vi "Jaxc_System.vi"() -> ()   [LabVIEW 2013]
uses:
  <vilib>/imath/engines/lvmath/Plug In/_Char/NIMS_CH_character datatype.ctl
  <instrlib>/niUSRP/niUSRP Fetch Rx Data (CDB).vi
  <vilib>/imath/engines/lvmath2/RunTimeEngine/NodeEndStatement/NIMS_NodeEndStatement_Output.vi
  <instcachedir>/0/NIMS_NodeEndStatement_Output_53EC0D466D134D7ABD903AC30B43404B.lvgen/NIMS_NodeEndStatement_Output_53EC0D466D134D7ABD903AC30B43404B_004.vi
  <vilib>/imath/engines/lvmath2/RunTimeEngine/ErrorHandling/NIMS_Finalize Error.vi
  <vilib>/imath/engines/lvmath2/RunTimeEngine/BuiltInFunctions/length/NIMS_length(GV).vi
  <instcachedir>/0/NIMS_length(GV)_08A3D13377FD4E4B96F5795FBF3698FA.lvgen/NIMS_length(GV)_08A3D13377FD4E4B96F5795FBF3698FA_001.vi
  <vilib>/imath/engines/lvmath2/RunTimeEngine/RangeToken/NIMS_Range_R2 - Integer.vi
  <instcachedir>/0/NIMS_Range_R2 - Integer_C51C130E5EA5464EA148B28CDAB9615A.lvgen/NIMS_Range_R2 - Integer_C51C130E5EA5464EA148B28CDAB9615A_000.vi
  <instcachedir>/0/NIMS_NodeEndStatement_Output_53EC0D466D134D7ABD903AC30B43404B.lvgen/NIMS_NodeEndStatement_Output_53EC0D466D134D7ABD903AC30B43404B_014.vi
  <instcachedir>/0/NIMS_NodeEndStatement_Output_53EC0D466D134D7ABD903AC30B43404B.lvgen/NIMS_NodeEndStatement_Output_53EC0D466D134D7ABD903AC30B43404B_011.vi
  <vilib>/imath/engines/lvmath2/RunTimeEngine/IndexRead/NIMS V(S).vi
  <instcachedir>/0/NIMS V(S)_0488751826AF41519A22953C041130DC.lvgen/NIMS V(S)_0488751826AF41519A22953C041130DC_005.vi
  <vilib>/imathl/engines/lvmath/Functions/Error Handling/Create Error.vi
  <vilib>/imath/engines/lvmath2/RunTimeEngine/BuiltInFunctions/abs/NIMS_abs(signed).vi
  <instcachedir>/0/NIMS_abs(signed)_C4FCB8E6058B49B797C7C8D53CA5F6EC.lvgen/NIMS_abs(signed)_C4FCB8E6058B49B797C7C8D53CA5F6EC_002.vi
  <vilib>/imath/engines/lvmath2/RunTimeEngine/Managers/WorkSpace/UID Generator.vi
  <vilib>/imath/engines/lvmath2/RunTimeEngine/Managers/SymbolTable/Clear UID.vi
  <instcachedir>/0/NIMS_NodeEndStatement_Output_53EC0D466D134D7ABD903AC30B43404B.lvgen/NIMS_NodeEndStatement_Output_53EC0D466D134D7ABD903AC30B43404B_000.vi
  <vilib>/imath/engines/lvmath2/RunTimeEngine/BuiltInFunctions/close/NIMS_close(Enums).vi
  <vilib>/imath/engines/lvmath2/RunTimeEngine/BuiltInFunctions/figure/NIMS_figure(I32).vi
  <vilib>/imath/engines/lvmath2/RunTimeEngine/BuiltInFunctions/plot/NIMS_plot(G, Str).vi
  <instcachedir>/0/NIMS_plot(G, Str)_30D49D8623E0484DBD39D394DDFCBE95.lvgen/NIMS_plot(G, Str)_30D49D8623E0484DBD39D394DDFCBE95_001.vi
  <vilib>/imath/engines/lvmath2/RunTimeEngine/BuiltInFunctions/crosscorr/NIMS_crosscorr(GV,GV,Str).vi
  <instcachedir>/0/NIMS_crosscorr(GV,GV,Str)_7F516622EB1B4986A7D0F3F178AC2F2E.lvgen/NIMS_crosscorr(GV,GV,Str)_7F516622EB1B4986A7D0F3F178AC2F2E_000.vi
  <instcachedir>/0/NIMS_abs(signed)_C4FCB8E6058B49B797C7C8D53CA5F6EC.lvgen/NIMS_abs(signed)_C4FCB8E6058B49B797C7C8D53CA5F6EC_006.vi
  <vilib>/imath/engines/lvmath2/RunTimeEngine/BuiltInFunctions/max/1 input/NIMS_max(RV).vi
  <instcachedir>/0/NIMS_max(RV)_237633DB1D604D5BA7001287DF3C7957.lvgen/NIMS_max(RV)_237633DB1D604D5BA7001287DF3C7957_000.vi
  <instcachedir>/0/NIMS_length(GV)_08A3D13377FD4E4B96F5795FBF3698FA.lvgen/NIMS_length(GV)_08A3D13377FD4E4B96F5795FBF3698FA_002.vi
  <vilib>/imath/engines/lvmath2/RunTimeEngine/IndexRead/NIMS V(R2).vi
  <instcachedir>/0/NIMS V(R2)_C76619605A0E4E9F8B2FA9389712AC47.lvgen/NIMS V(R2)_C76619605A0E4E9F8B2FA9389712AC47_001.vi
  <vilib>/imath/engines/lvmath2/RunTimeEngine/RunTimeType/NIMS_RunTimeType_From StrictType (excl LVString).vi
  <instcachedir>/0/NIMS_RunTimeType_From StrictType (excl LVString)_4DEE718D6EB74582AA20236969C084FC.lvgen/NIMS_RunTimeType_From StrictType (excl LVString)_4DEE718D6EB74582AA20236969C084FC_000.vi
  <vilib>/imath/engines/lvmath2/RunTimeEngine/LocalVariableDefStatement/MC_LocalVariableDefStatement_Display.vi
  <instcachedir>/0/NIMS_plot(G, Str)_30D49D8623E0484DBD39D394DDFCBE95.lvgen/NIMS_plot(G, Str)_30D49D8623E0484DBD39D394DDFCBE95_000.vi
  <vilib>/imath/engines/lvmath/Plug In/_Char/NIMS_CH_Character RV to String.vi
  <vilib>/imath/engines/lvmath2/RunTimeEngine/BuiltInFunctions/title/NIMS_title.vi
  <vilib>/imath/engines/lvmath2/RunTimeEngine/Managers/SymbolTable/NIMS_WorkSpace.lvlib
  <vilib>/imath/engines/lvmath2/RunTimeEngine/CommandStatement/MC_CommandStatement_break.vi
panel:
  out "error":i32
  in  "number of samples":i64=100000
  out "index_length":i32
  out "x_start":cdb[](array[numeric])
  out "a":cdb[](array[numeric])
  out "index":i32
  in  "stop 2":bool
  in  "RX number of samples":i64=100000
  out "RX coerced gain":dbl format="%#_6f"
  out "RX coerced IQ rate":dbl=100000.0 format="%#_6p"
  in  "RX gain":dbl format="%#_6f"
  in  "RX IQ rate":dbl=100000.0 format="%#_6p"
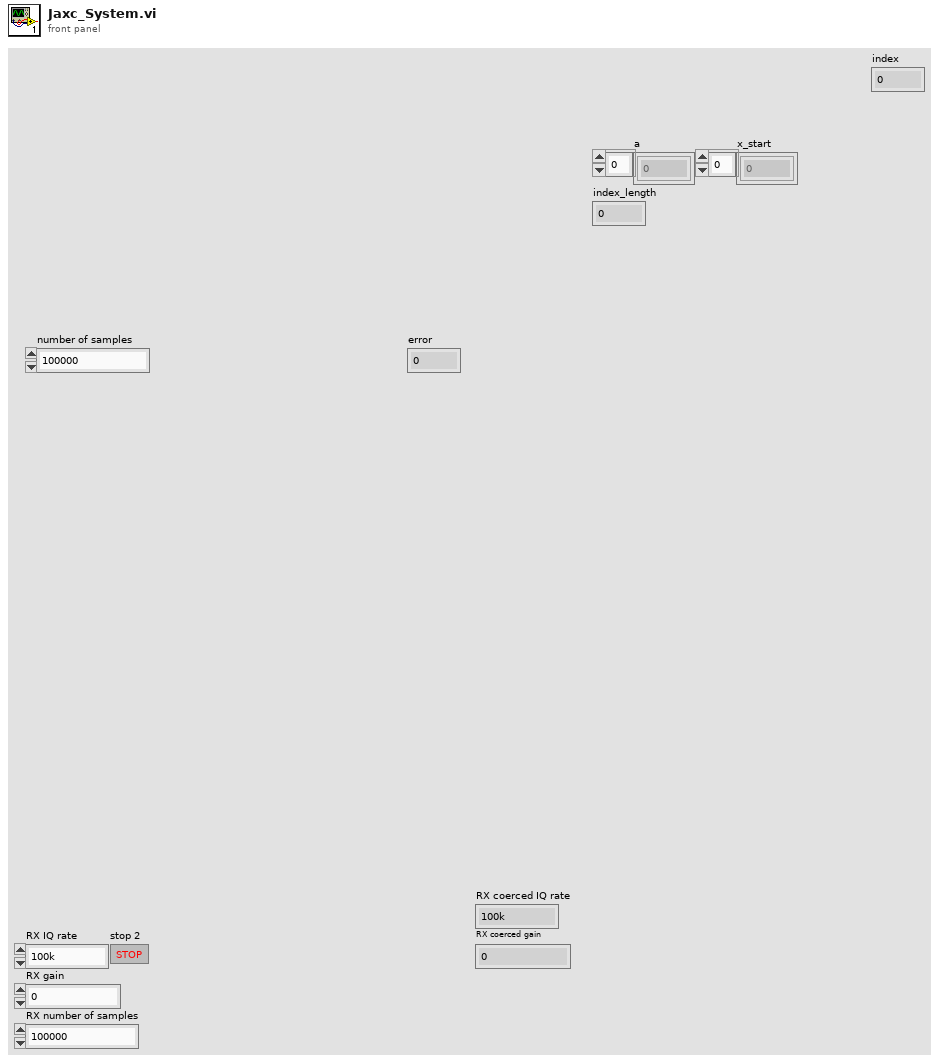
[diagram p1: front panel]
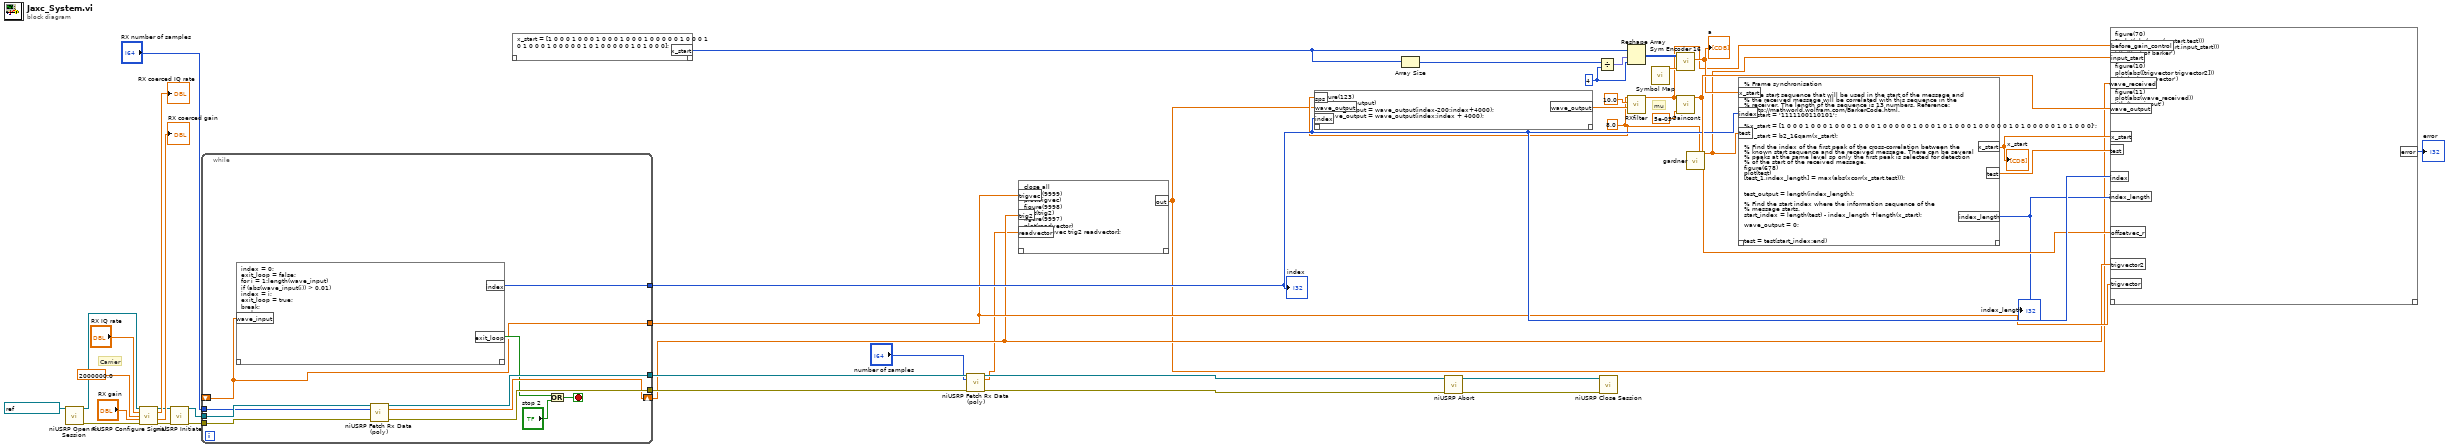
[diagram p0: block diagram]
diagram:
  w22 = 4 ("dimension size")
  w15 = 8.0 ("sps")
  # "mu"
  # "Carrier"
  n1 = call <instrlib>:"niUSRP Open Rx Session.vi"("device names"=refnum<k15> "192.168.10.9") -> ("session handle out"=w43:refnum<k15>, "error out"=w41:errorcluster)  [unwired: 13 in]
  n2 = call <instrlib>:"niUSRP Configure Signal.vi"("session handle"=w43, "IQ rate"="RX IQ rate", "carrier frequency"=2000000.0, "gain"="RX gain", "error in (no error)"=w41) -> ("session handle out"=w32:refnum<k15>, "coerced IQ rate"=→"RX coerced IQ rate":dbl, "coerced gain"=→"RX coerced gain":dbl, "error out"=w31:errorcluster)  [unwired: 6 in, 1 out]
  n3 = call <instrlib>:"niUSRP Initiate.vi"("session handle"=w32, "error in (no error)"=w31) -> ("session handle out"=w33:refnum<k15>, "error out"=w35:errorcluster)  [unwired: 12 in]
  n4 = while {
    tunnel: w33 -> [w55]
    tunnel: w35 -> [w54]
    tunnel: [w53] -> w11
    tunnel: [w52] -> w12
    tunnel: "RX number of samples" -> [w51]
    shift-right: [w50] -> w6
    shift-left: _ -> [w45]
    tunnel: [w49] -> w16
    tunnel: [w45] -> w7
    stop <- w47 stop-if-true
    n5 = mathscript code="index = 0;\nexit_loop = false;\nfor i = 1:length(wave_input)\nif (abs(wave_input(i)) > 0.01)\nindex = i;\nexit_loop = true;\nbreak;\nend\nend"("wave_input"=w45) -> ("index"=w49:i32, "exit_loop"=w46:bool)  [unwired: 1 in, 1 out]
    n6 = call-poly <instrlib>:"niUSRP Fetch Rx Data (poly).vi"("session handle"=w55, "number of samples"=w51, "error in (no error)"=w54) -> ("session handle out"=w53:refnum<k15>, "data"=w50:cdb[], "error out"=w52:errorcluster)  [unwired: 9 in, 1 out]
    n7 = Or(x=w46, y="stop 2") -> (x .or. y?=w47:bool)
  }
  "index" <- w16
  n8 = mathscript code="x_start = [1 0 0 0 1 0 0 0 1 0 0 0 1 0 0 0 1 0 0 0 0 0 1 0 0 0 1 0 1 0 0 0 1 0 0 0 0 0 1 0 1 0 0 0 0 0 1 0 1 0 0 0];"() -> ("x_start"=w1:i32[])  [unwired: 1 in, 1 out]
  n9 = call-poly <instrlib>:"niUSRP Fetch Rx Data (poly).vi"("session handle"=w11, "number of samples"="number of samples", "error in (no error)"=w12) -> ("session handle out"=w9:refnum<k15>, "data"=w5:cdb[], "error out"=w10:errorcluster)  [unwired: 9 in, 1 out]
  n10 = mathscript code="close all\nfigure(9999)\nplot(trigvec)\nfigure(9998)\nplot(trig2)\nfigure(9997)\nplot(readvector)\nout = [trigvec trig2 readvector];"("trigvec"=w7, "trig2"=w6, "readvector"=w5) -> ("out"=w4:cdb[])  [unwired: 1 in, 1 out]
  n11 = mathscript code="figure(123)\nplot(wave_output)\n%wave_output = wave_output(index-200:index+4000);\n%wave_output = wave_output(index:index + 4000);"("wave_output"=w4, "index"=w16, "sps"=w15) -> ("wave_output"=w27:cdb[])  [unwired: 1 in, 1 out]
  n12 = Array Size(array=w1) -> (size(s)=w20:i32)
  n13 = call <instrlib>:"niUSRP Abort.vi"("session handle"=w9, "error in (no error)"=w10) -> ("session handle out"=w42:refnum<k15>, "error out"=w40:errorcluster)  [unwired: 12 in]
  n14 = Divide(x=w20, y=w22) -> (x/y=w21:fxp<+,27,27>)
  n15 = call <instrlib>:"niUSRP Close Session.vi"("session handle"=w42, "error in (no error)"=w40) -> ()  [unwired: 13 in, 1 out]
  n16 = Reshape Array(w1, w21, w22) -> (w23:i32[][])
  n17 = call "RXfilter.vi"("Array"=w27, "span"=10.0, "sps"=w15) -> ("out"=w17:cdb[])  [unwired: 8 in]
  n18 = call "Symbol Map.vi"() -> ("symbol_map"=w24:cdb[])  [unwired: 11 in]
  n19 = call "Sym Encoder 16.vi"("symbol_map"=w24, "b"=w23) -> ("a"=w19:cdb[])  [unwired: 9 in]
  "a" <- w19
  n20 = call "Gaincont.vi"("mu"=5e-05, "Array"=w17) -> ("out"=w26:cdb[])  [unwired: 9 in]
  n21 = call "gardner.vi"("in"=w26, "sps"=w15) -> ("sym"=w3:cdb[], "offsetvec"=w14:dbl[])  [unwired: 12 in]
  n22 = mathscript code="% Frame synchronisation\n\n% The start sequence that will be used in the start of the message and\n% the received message will be correlated with this sequence in the \n% receiver. The length of the sequence is 13 numbers. Reference: \n% http://mathworld.wolfram.com/BarkerCode.html.\n%x_start = '1111100110101';\n\n%x_start = [1 0 0 0 1 0 0 0 1 0 0 0 1 0 0 0 1 0 0 0 0 0 1 0 0 0 1 0 1 0 0 0 1 0 0 0 0 0 1 0 1 0 0 0 0 0 1 0 1 0 0 0]';\n\n%x_start = b2_16qam(x_start);\n\n% Find the index of the first peak of the cross-correlation between the \n% known start sequence and the received message. There can be several \n% peaks at the same level so only the first peak is selected for detection \n% of the start of the received message.\nfigure(678)\nplot(test)\n[test_1,index_length] = max(abs(xcorr(x_start,test)));\n\n\ntest_output = length(index_length);\n\n% Find the start index where the information sequence of the \n% message starts.\nstart_index = length(test) - index_length +length(x_start);\n\nwave_output = 0;\n\n\ntest = test(start_index:end)"("test"=w3, "index"=w16, "x_start"=w19) -> ("test"=w25:cdb[], "x_start"=w18:cdb[], "index_length"=w13:i32)  [unwired: 1 in, 1 out]
  "x_start" <- w18
  "index_length" <- w13
  n23 = mathscript code="figure(70)\n%plot(abs(xcorr(x_start,test)))\nplot(abs(xcorr(x_start,input_start)))\ntitle('test of barker')\n\nfigure(10)\nplot(abs([trigvector trigvector2]))\ntitle('Trigger vector')\n\nfigure(11)\nplot(abs(wave_received))\ntitle('raw input')\nerror=10;"("wave_received"=w4, "wave_output"=w26, "test"=w25, "x_start"=w18, "input_start"=w3, "before_gain_control"=w17, "index"=w16, "offsetvec_r"=w14, "index_length"=w13, "trigvector"=w7, "trigvector2"=w6) -> ("error"=→"error":i32)  [unwired: 1 in, 1 out]
